vi "3.2.1_BOOST_Air_Muscle_Check.vi"(6 "Data in":T1, 8 "error in (no error)":errorcluster, 9 "AllControls In":T2, 10 "?":T3, 11 "Message Queue out":T4) -> (0 "error out":errorcluster, 1 "Flow":string, 2 "Data":T3, 3 "Message Queue Out":T4, 4 "Data out":T1)   [LabVIEW 2017]
uses:
  Depends/AMC/subVIs/TypeDefs/amc_Message Queue.ctl
  Depends/AMC/subVIs/TypeDefs/amc_Message.ctl
  Depends/Tools/Keyed Array/Tools_KeyedArray KeyedArray.ctl
  Ctrls/Data.ctl
  Ctrls/CSV_Data.ctl
  Ctrls/AllControls.ctl
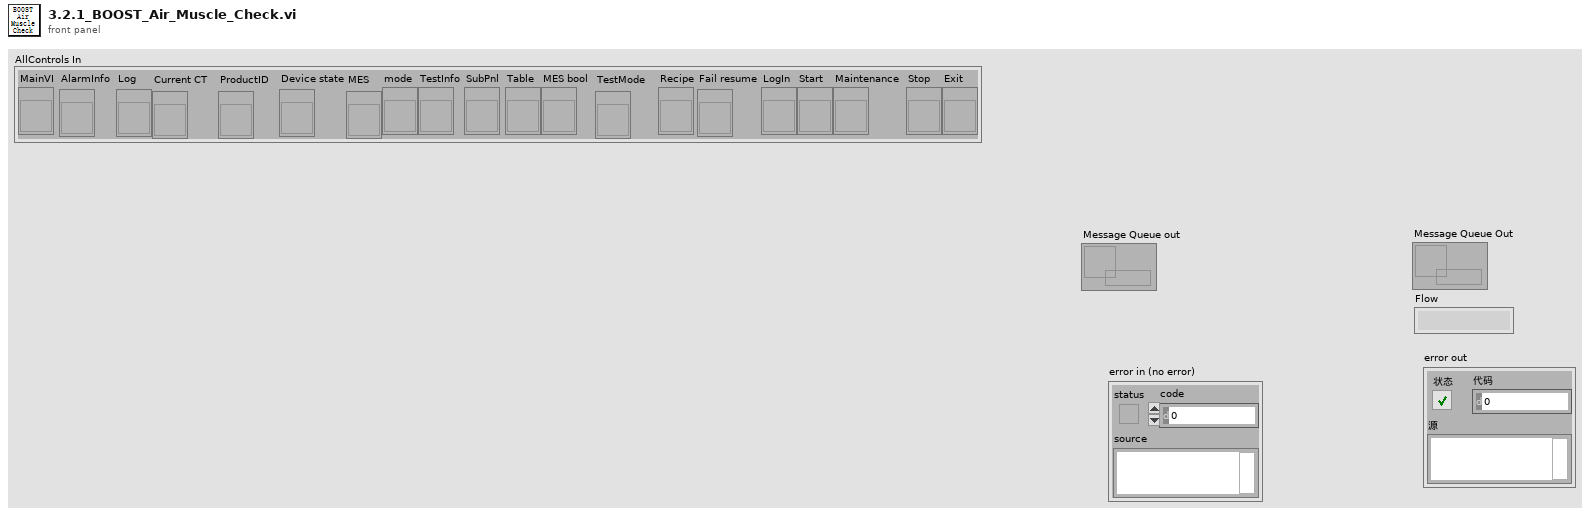
[diagram p1: front panel]
types:
  T1 = typedef "CSV_Data.ctl" = cluster{"Initialisation":cluster{"LMT - Connect UUT (con COM)":string, "LMT - Software Version (rrel)":string, "LMT - Write SKU file (wskuc)":string, "LMT - SKU file name":string, "Connect UUT DDM":string, "Read DDM EOL Timestamp - Mode":string, "Read DDM EOL Timestamp - Timestamp":string, "Read DDM EOL Timestamp - Rig ID":string, "Read DDM EOL Timestamp - Passmark ID":string, "Read DDM EOL Timestamp - Passmark Rev":string, "Software Version before flashing":string, "Read Hardware Serial":string, "UUT DDM SN":string, "Compare DDM SN with MES SN":string, "Backup PCBA Calibration EEPROM Response - CAL":string, "Flash Firmware Version":string, "Check SW Version":string, "Read DDM SW Version after flashing":string, "Set SKU Config":string, "Ready Status":string, "Set Device Mode to EOL":string, "DDM Parameter - Voltage":string, "DDM Parameter - Current":string, "DDM Parameter - Power":string, "DDM Parameter - Speed":string, "DDM Parameter - Pressure":string, "Tester Parameter - Voltage":string, "Tester Parameter - Current":string, "Tester Parameter - Power":string, "Tester Parameter - Ambient Pressure":string, "Tester Parameter - Ambient Temperature":string, "Calculated Parameter - DDM Pressure Corrected":string, "Calculated Parameter - DDM Real Power":string, "Calculated Parameter - Delta V":string}, "BEMF_Calibration":cluster{"Calibration Result - eol_cold_bemf_temp":string, "DDM Ambient Temp":string, "Restriction Plate Diameter":string, "Calibration Result - eol_bemf_mp_cold_coef_a":string, "Calibration Result - eol_bemf_mp_cold_coef_b":string, "Calibration Result - eol_bemf_mp_cold_coef_c":string, "Calibration Result - eol_bemf_lsi_cold_ref_coeffs":string, "Get - Calibration Result - eol_bemf_lsi_speed":string, "Get - Calibration Result - eol_bemf_lsi_integral_0":string, "Calibration Result - eol_bemf_lsi_integral_1":string, "Get - Calibration Result - eol_bemf_lsi_integral_2":string, "Get - Calibration Result - eol_cold_bemf":string, "Get - Calibration Result - eol_cold_bemf_fisf":string, "Finalise Calibration":string, "Compare -Calibration Result - eol_cold_bemf":string, "Compare -Calibration Result - eol_cold_bemf_fisf":string}, "ECO":cluster{"Reset Power Tune":string, "Reset BEMF FISF Calibration":string, "Restriction Plate Diameter":string, "ECO - Stabilisation Time":string, "ECO - DDM Parameter - Voltage":string, "ECO - DDM Parameter - Current":string, "ECO - DDM Parameter - Power":string, "ECO - DDM Parameter - Measured Power":string, "ECO - DDM Parameter - Speed":string, "ECO - DDM Parameter - Pressure":string, "ECO - Tester Parameter - Voltage":string, "ECO - Tester Parameter - Current":string, "ECO - Tester Parameter - Power":string, "ECO - Tester Parameter - Ambient Pressure":string, "ECO - Tester Parameter - Ambient Temperature":string, "ECO - Tester Parameter - Ambient Humidity":string, "ECO - Calculated Parameter - DDM Pressure Corrected":string, "ECO - Calculated Parameter - DDM Real Power":string, "ECO - Calculated Parameter - Delta V":string, "ECO - Calculated Parameter - Flowrate":string, "ECO - Calculated Parameter - Airwatt":string, "ECO - Formula":string, "PT ECO - Power Tune Mode Status":string}, "BOOST":cluster{"Restriction Plate Diameter":string, "BOOST - Stabilisation Time":string, "BOOST - DDM Parameter - Voltage":string, "BOOST - DDM Parameter - Current":string, "BOOST - DDM Parameter - Power":string, "BOOST - DDM Parameter - Measured Power":string, "BOOST - DDM Parameter - Speed":string, "BOOST - DDM Parameter - Pressure":string, "BOOST - Tester Parameter - Voltage":string, "BOOST - Tester Parameter - Current":string, "BOOST - Tester Parameter - Power":string, "BOOST - Tester Parameter - Ambient Pressure":string, "BOOST - Tester Parameter - Ambient Temperature":string, "BOOST - Tester Parameter - Ambient Humidity":string, "BOOST - Calculated Parameter - DDM Pressure Corrected":string, "BOOST - Calculated Parameter - DDM Real Power":string, "BOOST - Calculated Parameter - Delta V":string, "BOOST - Calculated Parameter - Flowrate":string, "BOOST - Calculated Parameter - Airwatt":string, "BOOST - Get AM Presence":string, "Air Muscle Turn Off Status":string, "BOOST - Air Muscle Calculated Parameter - Airwatt B":string, "BOOST - Air Muscle Calculate Airwatt Delta":string, "PT BOOST - Power Tune Mode Status":string, "Finalise Calibration":string, "ECO - Get AW Calibration value":string, "BOOST - Get AW Calibration value":string}, "MAX":cluster{"Restriction Plate Diameter":string, "MAX - Stabilisation Time":string, "Get Average Delta Tmag (LSIdelta_FISFdelta_LSItmag_FISFtmag_IIRtmag)":string, "Get Average Delta Tmag FISF":string, "MAX - DDM Parameter - Voltage":string, "MAX - DDM Parameter - Current":string, "MAX - DDM Parameter - Power":string, "MAX - DDM Parameter - Measured Power":string, "MAX - DDM Parameter - Speed":string, "MAX - DDM Parameter - Pressure":string, "MAX - Tester Parameter - Voltage":string, "MAX - Tester Parameter - Current":string, "MAX - Tester Parameter - Power":string, "MAX - Tester Parameter - Ambient Pressure":string, "MAX - Tester Parameter - Ambient Temperature":string, "MAX - Tester Parameter - Ambient Humidity":string, "MAX - Calculated Parameter - DDM Pressure Corrected":string, "MAX - Calculated Parameter - DDM Real Power":string, "MAX - Calculated Parameter - Delta V":string, "MAX - Calculated Parameter - Flowrate":string, "MAX - Calculated Parameter - Airwatt":string, "MAX_FISF_Check_Average_Delta_Tmag":string, "MAX - FISF - BEMF Finetune Result":string, "MAX tune - Delta P1":string, "MAX tune - Calculated Parameter - Airwatt":string, "Calculate Delta Airwatts - MAX finetune - Delta P2":string, "MAX finetune - DDM Parameter - Voltage":string, "MAX finetune - DDM Parameter - Current":string, "MAX finetune - DDM Parameter - Power":string, "MAX finetune - DDM Parameter - Measured Power":string, "MAX finetune - DDM Parameter - Speed":string, "MAX finetune - DDM Parameter - Pressure":string, "MAX finetune - Tester Parameter - Voltage":string, "MAX finetune - Tester Parameter - Current":string, "MAX finetune - Tester Parameter - Power":string, "MAX finetune - Tester Parameter - Ambient Pressure":string, "MAX finetune - Tester Parameter - Ambient Temperature":string, "MAX finetune - Tester Parameter - Ambient Humidity":string, "MAX finetune - Calculated Parameter - DDM Pressure Corrected":string, "MAX finetune - Calculated Parameter - DDM Real Power":string, "MAX finetune - Calculated Parameter - Delta V":string, "MAX finetune - Calculated Parameter - Flowrate":string, "MAX finetune - Calculated Parameter - Airwatt":string, "Check Derate Result":string, "Delta Tmag FISF":string, "Get Hot BEMF Result":string, "Calculate delta Pressure":string, "Finalise Calibration":string, "Calculate & Check Delta BEMF":string, "Delta P Airwatts Value":string}, "LL":cluster{"DDM Ambient Temp":string, "Restriction Plate Diameter":string, "LL - DDM Parameter - Voltage":string, "LL - DDM Parameter - Current":string, "LL - DDM Parameter - Power":string, "LL - DDM Parameter - Measured Power":string, "LL - DDM Parameter - Speed":string, "LL - DDM Parameter - Pressure":string, "LL - Tester Parameter - Voltage":string, "LL - Tester Parameter - Current":string, "LL - Tester Parameter - Power":string, "LL - DDM Real Power":string, "LL - Calibrate Task Detect LL":string}, "HL":cluster{"HL - DDM Parameter - Voltage":string, "HL - DDM Parameter - Current":string, "HL - DDM Parameter - Power":string, "HL - DDM Parameter - Measured Power":string, "HL - DDM Parameter - Speed":string, "HL - DDM Parameter - Pressure":string, "HL - Tester Parameter - Voltage":string, "HL - Tester Parameter - Current":string, "HL - Tester Parameter - Power":string, "HL - DDM Real Power":string, "HL - Calibrate Task Detect HL":string}, "LH":cluster{"Restriction Plate Diameter":string, "LH - DDM Parameter - Voltage":string, "LH - DDM Parameter - Current":string, "LH - DDM Parameter - Power":string, "LH - DDM Parameter - Measured Power":string, "LH - DDM Parameter - Speed":string, "LH - DDM Parameter - Pressure":string, "LH - Tester Parameter - Voltage":string, "LH - Tester Parameter - Current":string, "LH - Tester Parameter - Power":string, "LH - DDM Real Power":string, "LH - Calibrate Task Detect LH":string}, "HH":cluster{"HH - DDM Parameter - Voltage":string, "HH - DDM Parameter - Current":string, "HH - DDM Parameter - Power":string, "HH - DDM Parameter - Measured Power":string, "HH - DDM Parameter - Speed":string, "HH - DDM Parameter - Pressure":string, "HH - Tester Parameter - Voltage":string, "HH - Tester Parameter - Current":string, "HH - Tester Parameter - Power":string, "HH - DDM Real Power":string, "HH - Calibrate Task Detect HH":string}, "Inlet Blockage Calibration":cluster{"Inlet Blockage Calibration - DDM Parameter - Voltage":string, "Inlet Blockage Calibration - DDM Parameter - Current":string, "Inlet Blockage Calibration - DDM Parameter - Power":string, "Inlet Blockage Calibration - DDM Parameter - Measured Power":string, "Inlet Blockage Calibration - DDM Parameter - Speed":string, "Inlet Blockage Calibration - DDM Parameter - Pressure":string, "Inlet Blockage Calibration - Tester Parameter - Voltage":string, "Inlet Blockage Calibration - Tester Parameter - Current":string, "Inlet Blockage Calibration - Tester Parameter - Power":string, "Inlet Blockage Calibration - DDM Real Power":string, "Calibration Inlet Blockage_E":string, "Finalise Calibration":string, "Get Task Detect LL":string, "Get Task Detect HL":string, "Get Task Detect LH":string, "Get Task Detect HH":string, "Calibration Inlet Blockage":string, "Calibration eol cold bemf temp":string}, "GOOD":cluster{"GOOD UNIT - Clear EEPROM Error Log":string, "GOOD UNIT - Write Product Timestamp - Mode":string, "GOOD UNIT - Write Product Timestamp - Timestamp":string, "GOOD UNIT - Write Product Timestamp - Rig ID":string, "GOOD UNIT - Write Product Timestamp - Passmark ID":string, "GOOD UNIT - Write Product Timestamp - Passmark Rev":string, "GOOD UNIT - Set Device Mode to PROD":string, "GOOD UNIT - Backup PCBA Calibration EEPROM Response":string, "GOOD UNIT - Check Security Bit":string, "GOOD UNIT - Set Calibration Lock":string, "GOOD UNIT - Get_Calibration_Lock":string, "GOOD UNIT - Disconnect UUT":string}, "NG":cluster{"NG UNIT - Read NVM Error":string, "NG UNIT - Set Device Mode to FCT":string, "NG UNIT - Backup PCBA Calibration EEPROM Response - CAL":string, "NG UNIT - Backup PCBA Calibration EEPROM Response - ERROR":string, "NG UNIT - Backup PCBA Calibration EEPROM Response - USAGE":string, "NG UNIT - Disconnect UUT":string}, "SN":string, "Table":string[][], "Count":cluster{"Total":i32, "OK":i32, "NG":i32, "Yield":dbl}, "Start Time":timestamp, "daemon reference":refnum<k5>, "CT":dbl, "Config":string[][], "OK/NG":bool, "Station ID":string, "MES DDM SN":string, "MES PCBA SN":string, "Retest":string, "Lux":string, "Initialisation_Status":cluster{"LMT - Connect UUT (con COM)":string, "LMT - Software Version (rrel)":string, "LMT - Write SKU file (wskuc)":string, "LMT - SKU file name":string, "Connect UUT DDM":string, "Read DDM EOL Timestamp - Mode":string, "Read DDM EOL Timestamp - Timestamp":string, "Read DDM EOL Timestamp - Rig ID":string, "Read DDM EOL Timestamp - Passmark ID":string, "Read DDM EOL Timestamp - Passmark Rev":string, "Software Version before flashing":string, "Read Hardware Serial":string, "UUT DDM SN":string, "Compare DDM SN with MES SN":string, "Backup PCBA Calibration EEPROM Response - CAL":string, "Flash Firmware Version":string, "Check SW Version":string, "Read DDM SW Version after flashing":string, "Set SKU Config":string, "Ready Status":string, "Set Device Mode to EOL":string, "DDM Parameter - Voltage":string, "DDM Parameter - Current":string, "DDM Parameter - Power":string, "DDM Parameter - Speed":string, "DDM Parameter - Pressure":string, "Tester Parameter - Voltage":string, "Tester Parameter - Current":string, "Tester Parameter - Power":string, "Tester Parameter - Ambient Pressure":string, "Tester Parameter - Ambient Temperature":string, "Calculated Parameter - DDM Pressure Corrected":string, "Calculated Parameter - DDM Real Power":string, "Calculated Parameter - Delta V":string}, "BEMF_Calibration_Status":cluster{"Calibration Result - eol_cold_bemf_temp":string, "DDM Ambient Temp":string, "Restriction Plate Diameter":string, "Calibration Result - eol_bemf_mp_cold_coef_a":string, "Calibration Result - eol_bemf_mp_cold_coef_b":string, "Calibration Result - eol_bemf_mp_cold_coef_c":string, "Calibration Result - eol_bemf_lsi_cold_ref_coeffs":string, "Get - Calibration Result - eol_bemf_lsi_speed":string, "Get - Calibration Result - eol_bemf_lsi_integral_0":string, "Calibration Result - eol_bemf_lsi_integral_1":string, "Get - Calibration Result - eol_bemf_lsi_integral_2":string, "Get - Calibration Result - eol_cold_bemf":string, "Get - Calibration Result - eol_cold_bemf_fisf":string, "Finalise Calibration":string, "Compare -Calibration Result - eol_cold_bemf":string, "Compare -Calibration Result - eol_cold_bemf_fisf":string}, "ECO_Status":cluster{"Reset Power Tune":string, "Reset BEMF FISF Calibration":string, "Restriction Plate Diameter":string, "ECO - Stabilisation Time":string, "ECO - DDM Parameter - Voltage":string, "ECO - DDM Parameter - Current":string, "ECO - DDM Parameter - Power":string, "ECO - DDM Parameter - Measured Power":string, "ECO - DDM Parameter - Speed":string, "ECO - DDM Parameter - Pressure":string, "ECO - Tester Parameter - Voltage":string, "ECO - Tester Parameter - Current":string, "ECO - Tester Parameter - Power":string, "ECO - Tester Parameter - Ambient Pressure":string, "ECO - Tester Parameter - Ambient Temperature":string, "ECO - Tester Parameter - Ambient Humidity":string, "ECO - Calculated Parameter - DDM Pressure Corrected":string, "ECO - Calculated Parameter - DDM Real Power":string, "ECO - Calculated Parameter - Delta V":string, "ECO - Calculated Parameter - Flowrate":string, "ECO - Calculated Parameter - Airwatt":string, "ECO - Formula":string, "PT ECO - Power Tune Mode Status":string}, "BOOST_Status":cluster{"Restriction Plate Diameter":string, "BOOST - Stabilisation Time":string, "BOOST - DDM Parameter - Voltage":string, "BOOST - DDM Parameter - Current":string, "BOOST - DDM Parameter - Power":string, "BOOST - DDM Parameter - Measured Power":string, "BOOST - DDM Parameter - Speed":string, "BOOST - DDM Parameter - Pressure":string, "BOOST - Tester Parameter - Voltage":string, "BOOST - Tester Parameter - Current":string, "BOOST - Tester Parameter - Power":string, "BOOST - Tester Parameter - Ambient Pressure":string, "BOOST - Tester Parameter - Ambient Temperature":string, "BOOST - Tester Parameter - Ambient Humidity":string, "BOOST - Calculated Parameter - DDM Pressure Corrected":string, "BOOST - Calculated Parameter - DDM Real Power":string, "BOOST - Calculated Parameter - Delta V":string, "BOOST - Calculated Parameter - Flowrate":string, "BOOST - Calculated Parameter - Airwatt":string, "BOOST - Get AM Presence":string, "Air Muscle Turn Off Status":string, "BOOST - Air Muscle Calculated Parameter - Airwatt B":string, "BOOST - Air Muscle Calculate Airwatt Delta":string, "PT BOOST - Power Tune Mode Status":string, "Finalise Calibration":string, "ECO - Get AW Calibration value":string, "BOOST - Get AW Calibration value":string}, "MAX_Status":cluster{"Restriction Plate Diameter":string, "MAX - Stabilisation Time":string, "Get Average Delta Tmag (LSIdelta_FISFdelta_LSItmag_FISFtmag_IIRtmag)":string, "Get Average Delta Tmag FISF":string, "MAX - DDM Parameter - Voltage":string, "MAX - DDM Parameter - Current":string, "MAX - DDM Parameter - Power":string, "MAX - DDM Parameter - Measured Power":string, "MAX - DDM Parameter - Speed":string, "MAX - DDM Parameter - Pressure":string, "MAX - Tester Parameter - Voltage":string, "MAX - Tester Parameter - Current":string, "MAX - Tester Parameter - Power":string, "MAX - Tester Parameter - Ambient Pressure":string, "MAX - Tester Parameter - Ambient Temperature":string, "MAX - Tester Parameter - Ambient Humidity":string, "MAX - Calculated Parameter - DDM Pressure Corrected":string, "MAX - Calculated Parameter - DDM Real Power":string, "MAX - Calculated Parameter - Delta V":string, "MAX - Calculated Parameter - Flowrate":string, "MAX - Calculated Parameter - Airwatt":string, "MAX_FISF_Check_Average_Delta_Tmag":string, "MAX - FISF - BEMF Finetune Result":string, "MAX tune - Delta P1":string, "MAX tune - Calculated Parameter - Airwatt":string, "Calculate Delta Airwatts - MAX finetune - Delta P2":string, "MAX finetune - DDM Parameter - Voltage":string, "MAX finetune - DDM Parameter - Current":string, "MAX finetune - DDM Parameter - Power":string, "MAX finetune - DDM Parameter - Measured Power":string, "MAX finetune - DDM Parameter - Speed":string, "MAX finetune - DDM Parameter - Pressure":string, "MAX finetune - Tester Parameter - Voltage":string, "MAX finetune - Tester Parameter - Current":string, "MAX finetune - Tester Parameter - Power":string, "MAX finetune - Tester Parameter - Ambient Pressure":string, "MAX finetune - Tester Parameter - Ambient Temperature":string, "MAX finetune - Tester Parameter - Ambient Humidity":string, "MAX finetune - Calculated Parameter - DDM Pressure Corrected":string, "MAX finetune - Calculated Parameter - DDM Real Power":string, "MAX finetune - Calculated Parameter - Delta V":string, "MAX finetune - Calculated Parameter - Flowrate":string, "MAX finetune - Calculated Parameter - Airwatt":string, "Check Derate Result":string, "Delta Tmag FISF":string, "Get Hot BEMF Result":string, "Calculate delta Pressure":string, "Finalise Calibration":string, "Calculate & Check Delta BEMF":string, "Delta P Airwatts Value":string}, "LL_Status":cluster{"DDM Ambient Temp":string, "Restriction Plate Diameter":string, "LL - DDM Parameter - Voltage":string, "LL - DDM Parameter - Current":string, "LL - DDM Parameter - Power":string, "LL - DDM Parameter - Measured Power":string, "LL - DDM Parameter - Speed":string, "LL - DDM Parameter - Pressure":string, "LL - Tester Parameter - Voltage":string, "LL - Tester Parameter - Current":string, "LL - Tester Parameter - Power":string, "LL - DDM Real Power":string, "LL - Calibrate Task Detect LL":string}, "HL_Status":cluster{"HL - DDM Parameter - Voltage":string, "HL - DDM Parameter - Current":string, "HL - DDM Parameter - Power":string, "HL - DDM Parameter - Measured Power":string, "HL - DDM Parameter - Speed":string, "HL - DDM Parameter - Pressure":string, "HL - Tester Parameter - Voltage":string, "HL - Tester Parameter - Current":string, "HL - Tester Parameter - Power":string, "HL - DDM Real Power":string, "HL - Calibrate Task Detect HL":string}, "LH_Status":cluster{"Restriction Plate Diameter":string, "LH - DDM Parameter - Voltage":string, "LH - DDM Parameter - Current":string, "LH - DDM Parameter - Power":string, "LH - DDM Parameter - Measured Power":string, "LH - DDM Parameter - Speed":string, "LH - DDM Parameter - Pressure":string, "LH - Tester Parameter - Voltage":string, "LH - Tester Parameter - Current":string, "LH - Tester Parameter - Power":string, "LH - DDM Real Power":string, "LH - Calibrate Task Detect LH":string}, "HH_Status":cluster{"HH - DDM Parameter - Voltage":string, "HH - DDM Parameter - Current":string, "HH - DDM Parameter - Power":string, "HH - DDM Parameter - Measured Power":string, "HH - DDM Parameter - Speed":string, "HH - DDM Parameter - Pressure":string, "HH - Tester Parameter - Voltage":string, "HH - Tester Parameter - Current":string, "HH - Tester Parameter - Power":string, "HH - DDM Real Power":string, "HH - Calibrate Task Detect HH":string}, "Inlet Blockage Calibration_Status":cluster{"Inlet Blockage Calibration - DDM Parameter - Voltage":string, "Inlet Blockage Calibration - DDM Parameter - Current":string, "Inlet Blockage Calibration - DDM Parameter - Power":string, "Inlet Blockage Calibration - DDM Parameter - Measured Power":string, "Inlet Blockage Calibration - DDM Parameter - Speed":string, "Inlet Blockage Calibration - DDM Parameter - Pressure":string, "Inlet Blockage Calibration - Tester Parameter - Voltage":string, "Inlet Blockage Calibration - Tester Parameter - Current":string, "Inlet Blockage Calibration - Tester Parameter - Power":string, "Inlet Blockage Calibration - DDM Real Power":string, "Calibration Inlet Blockage_E":string, "Finalise Calibration":string, "Get Task Detect LL":string, "Get Task Detect HL":string, "Get Task Detect LH":string, "Get Task Detect HH":string, "Calibration Inlet Blockage":string, "Calibration eol cold bemf temp":string}, "GOOD_Status":cluster{"GOOD UNIT - Clear EEPROM Error Log":string, "GOOD UNIT - Write Product Timestamp - Mode":string, "GOOD UNIT - Write Product Timestamp - Timestamp":string, "GOOD UNIT - Write Product Timestamp - Rig ID":string, "GOOD UNIT - Write Product Timestamp - Passmark ID":string, "GOOD UNIT - Write Product Timestamp - Passmark Rev":string, "GOOD UNIT - Set Device Mode to PROD":string, "GOOD UNIT - Backup PCBA Calibration EEPROM Response":string, "GOOD UNIT - Check Security Bit":string, "GOOD UNIT - Set Calibration Lock":string, "GOOD UNIT - Get_Calibration_Lock":string, "GOOD UNIT - Disconnect UUT":string}, "NG_Status":cluster{"NG UNIT - Read NVM Error":string, "NG UNIT - Set Device Mode to FCT":string, "NG UNIT - Backup PCBA Calibration EEPROM Response - CAL":string, "NG UNIT - Backup PCBA Calibration EEPROM Response - ERROR":string, "NG UNIT - Backup PCBA Calibration EEPROM Response - USAGE":string, "NG UNIT - Disconnect UUT":string}, "SKU":string, "Plate_Diameter":string, "Alarm":string}
  T2 = typedef "AllControls.ctl" = cluster{"MainVI":refnum<vi>, "AlarmInfo":refnum<vi>, "Log":refnum<vi>, "Current CT":refnum<vi>, "ProductID":refnum<vi>, "Device state":refnum<vi>, "MES":refnum<vi>, "mode":refnum<vi>, "TestInfo":refnum<vi>, "SubPnl":refnum<vi>, "Table":refnum<vi>, "MES bool":refnum<vi>, "TestMode":refnum<vi>, "Recipe":refnum<vi>, "Fail resume":refnum<vi>, "LogIn":refnum<vi>, "Start":refnum<vi>, "Maintenance":refnum<vi>, "Stop":refnum<vi>, "Exit":refnum<vi>}
  T3 = typedef "Data.ctl" = cluster{"Initialisation":cluster{"DDM_Parameter":dbl[], "DDM_Parameter_status":bool[], "Get_Tester_Parameter":dbl[], "Get_Tester_Parameter_status":bool[], "Cal_Tester_Parameter":dbl[], "Cal_Tester_Parameter_status":bool[], "sw_version_before_status":bool, "sw_version_after_status":bool, "Set_SKU_Config_With_LMT_status":bool, "FCT_timestamp_status":bool, "LMT_Connect_to_UUT_status":bool}, "BEMF_Calibration":cluster{"Read_ambient_temperature":dbl, "Calibration_Vaule":dbl[], "Calibration_Vaule _B":dbl[], "Calibration_Vaule_status":bool[], "Calibration_Vaule_B_status":bool[]}, "ECO":cluster{"DDM_Parameter":dbl[], "DDM_Parameter_status":bool[], "Get_Tester_Parameter":dbl[], "Get_Tester_Parameter_status":bool[], "Cal_Tester_Parameter":dbl[], "Cal_Tester_Parameter_status":bool[], "DDM_Parameter_after_power_tune":dbl[], "Get_Tester_Parameter_after_power_tune":dbl[], "Cal_Tester_Parameter_after_power_tune":dbl[], "Cal_Tester_Parameter_after_power_tune_status":bool[], "Delta_P":dbl}, "BOOST":cluster{"DDM_Parameter":dbl[], "DDM_Parameter_status":bool[], "Get_Tester_Parameter":dbl[], "Get_Tester_Parameter_status":bool[], "Cal_Tester_Parameter":dbl[], "Cal_Tester_Parameter_status":bool[], "DDM_Parameter_after_power_tune":dbl[], "Get_Tester_Parameter_after_power_tune":dbl[], "Cal_Tester_Parameter_after_power_tune":dbl[], "Cal_Tester_Parameter_after_power_tune_status":bool[], "airwatts_am_off":dbl, "AW_Delta_(AM_on_and_off)":dbl, "AW_Delta_(AM_on_and_off)_Status":bool, "Delta_P":dbl}, "MAX":cluster{"Average_Tmag_Data":cluster{"LSI Delta in degC":dbl, "FISF Delta in degc":dbl, "LSI Tmag in degC":dbl, "Fisf Tmag in degC":dbl, "IIR Tmag in degC":dbl}, "DDM_Parameter":dbl[], "DDM_Parameter_status":bool[], "Get_Tester_Parameter":dbl[], "Get_Tester_Parameter_status":bool[], "Cal_Tester_Parameter":dbl[], "BEMF_Finetune":cluster{"eol_bemf_mp_cold_coef_c":dbl, "eol_cold_bemf_fisf_offset":dbl}, "AW_Tune":cluster{"delta_P1":dbl, "delta_P_Setting":dbl}, "DDM_Parameter_after_Airwatts_Tune":dbl[], "Get_Tester_Parameter_after_Airwatts_Tune":dbl[], "Cal_Tester_Parameter_after_Airwatts_Tune":dbl[], "DDM_Parameter_after_Airwatts_Finetune":dbl[], "Get_Tester_Parameter_after_Airwatts_Finetune":dbl[], "Cal_Tester_Parameter_after_Airwatts_Finetune":dbl[], "AW_Finetune":cluster{"delta_P2":dbl, "delta_P_Setting":dbl}, "Delta_Tmag_after_tune":cluster{"LSI Delta in degC":dbl, "FISF Delta in degc":dbl, "LSI Tmag in degC":dbl, "Fisf Tmag in degC":dbl, "IIR Tmag in degC":dbl}, "Hot Bemf in mV":dbl, "DDM_Pressure":dbl, "Delta_Pressure":dbl, " Cold Bemf in mV":dbl, " delta Bemf":dbl, " delta p":dbl, "Delta_Pressure_status":bool, " delta Bemf_status":bool, "LSI Delta in degC_status":bool, "FISF Delta in degc_status":bool, "Max_check_derate_status_status":bool, "Average_All_data":dbl[][], "Average_Tmag_Data_status":bool[], "Average_Tmag_Data_after_tune_status":bool[], "Cal_Tester_Parameter_status":bool[], "Cal_Tester_Parameter_status_after_Airwatts_Tune":bool[], "Cal_Tester_Parameter_status_after_Airwatts_FineTune":bool[]}, "Task_Detect_Calib":cluster{"LL":cluster{"DDM_Parameter":dbl[], "DDM_Parameter_status":bool[], "Get_Tester_Parameter":dbl[], "Get_Tester_Parameter_status":bool[], "Set_task_detect_A":dbl, "Set_task_detect_A_Status":bool}, "HL":cluster{"DDM_Parameter":dbl[], "DDM_Parameter_status":bool[], "Get_Tester_Parameter":dbl[], "Get_Tester_Parameter_status":bool[], "Set_task_detect_B":dbl, "Set_task_detect_B_Status":bool}, "LH":cluster{"DDM_Parameter":dbl[], "DDM_Parameter_status":bool[], "Get_Tester_Parameter":dbl[], "Get_Tester_Parameter_status":bool[], "Set_task_detect_C":dbl, "Set_task_detect_C_Status":bool}, "HH":cluster{"DDM_Parameter":dbl[], "DDM_Parameter_status":bool[], "Get_Tester_Parameter":dbl[], "Get_Tester_Parameter_status":bool[], "Set_task_detect_D":dbl, "Read_and_check_calibration_Status":bool[], "Set_task_detect_D_Status":bool}, "Get_eol_inlet_blockage_E":dbl, "Calib_vaule":cluster{"Get_task_detect_LL":dbl, "Get_task_detect_HL":dbl, "Get_task_detect_LH":dbl, "Get_task_detect_HH":dbl, "eol_inlet_blockage":dbl, "eol_code_bemf_temp":dbl}, "calibrated temp":dbl, "Inlet_Blockage_Calibration":cluster{"DDM_Parameter":dbl[], "DDM_Parameter_status":bool[], "Get_Tester_Parameter":dbl[], "Get_Tester_Parameter_status":bool[]}, "Get_eol_inlet_blockage_E_Status":bool}, "good":cluster{"Write_Product_TS":cluster{"TIMESTAMP":i64, "RIG_ID":i64, "PASSMARK_ID":i64, "PASSMARK_REV":i64}, "Read_Product_TS":cluster{"TIMESTAMP":i64, "RIG_ID":i64, "PASSMARK_ID":i64, "PASSMARK_REV":i64}, "Good_Check_Secuity_Bit_Stauts":bool}}
  T4 = typedef "amc_Message Queue.ctl" = refnum<queue>
  T5 = typedef "HD Config.ctl" = cluster{" PC":cluster{"PC Address":u8[], "PC Port":i32}, "FCO":cluster{"COM":refnum<visa-resource-name>, "Baudrate":u32}, "DC Power ":cluster{"COM":refnum<visa-resource-name>, "Baudrate":u32}, "PW3336":cluster{"COM":refnum<visa-resource-name>, "Baudrate":u32}, "Lefoo":cluster{"COM":refnum<visa-resource-name>, "Baudrate":u32}, "Tempt&Hum":cluster{"COM":refnum<visa-resource-name>, "Baudrate":u32}, "DIPC":cluster{"COM":refnum<visa-resource-name>}, "Daemon":cluster{"IP Address":string, "Port":u16, "Retry":u16}, "NFC":cluster{"COM":refnum<visa-resource-name>, "Baudrate":u32}, "Fail_resume_mode":bool, "GRR":bool}
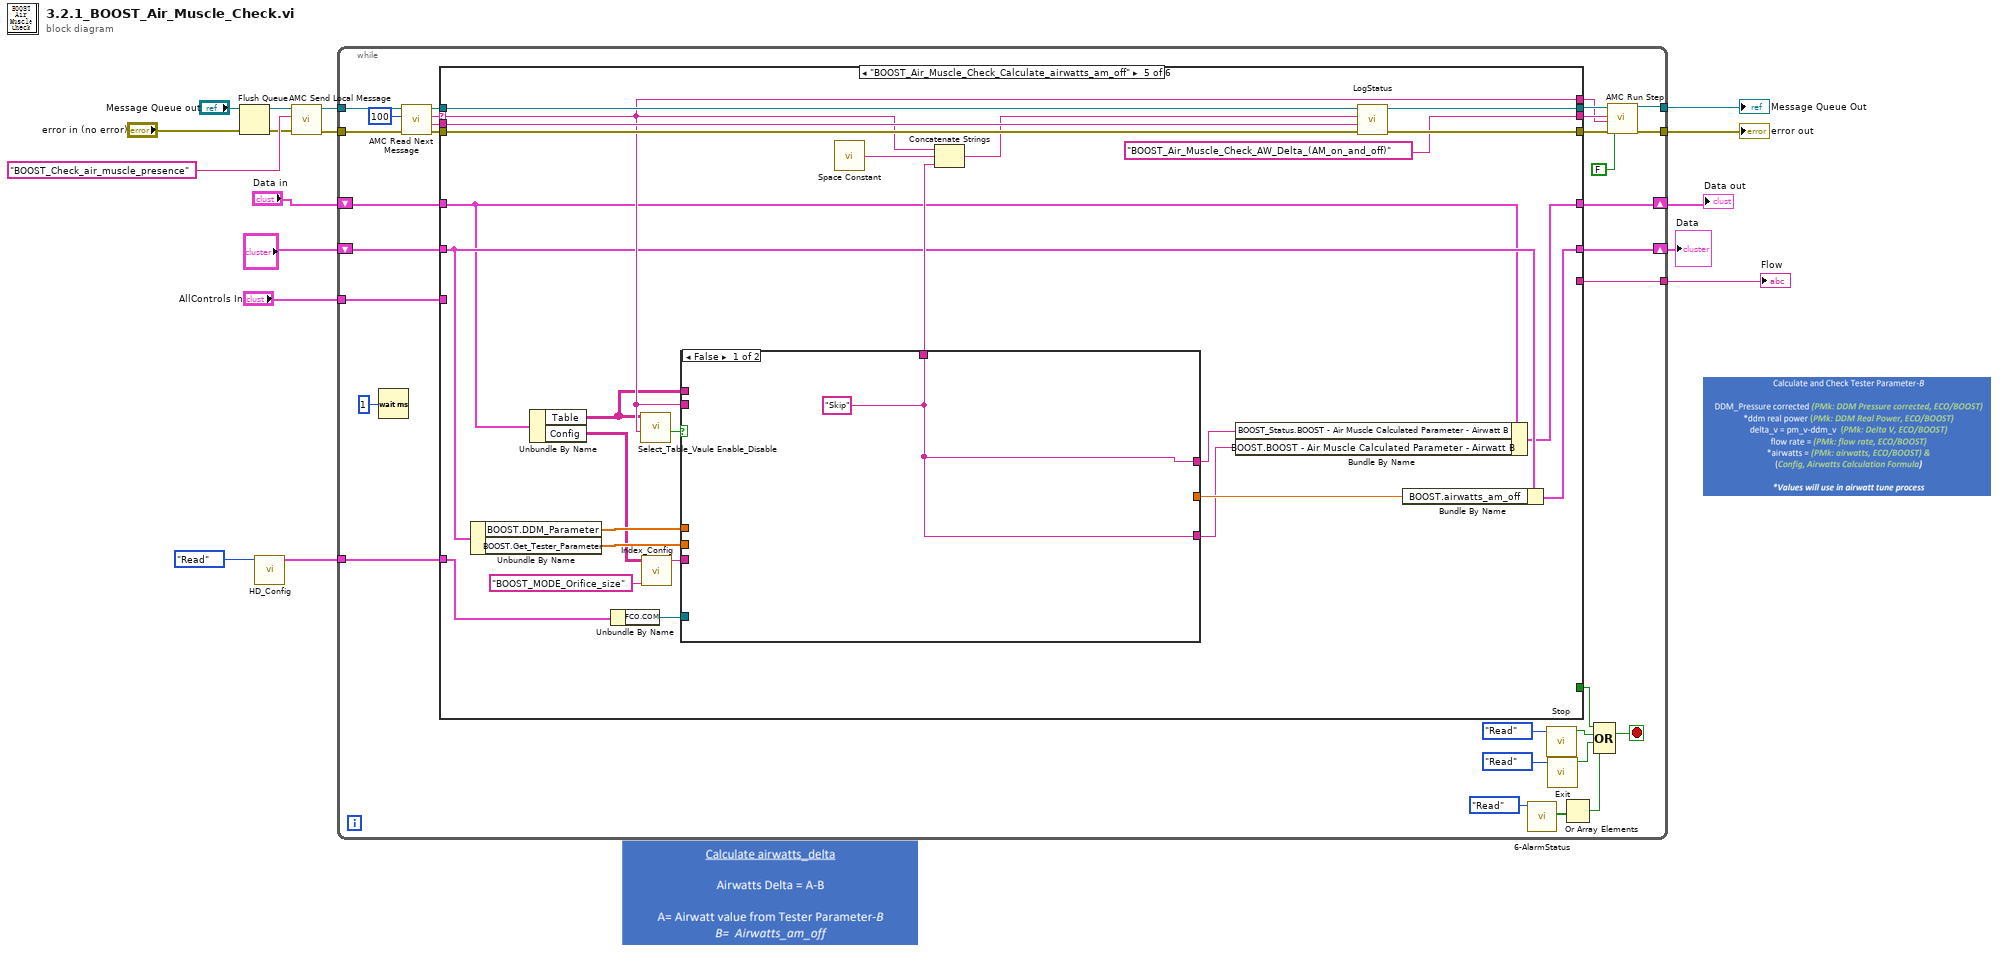
[diagram p0: block diagram]
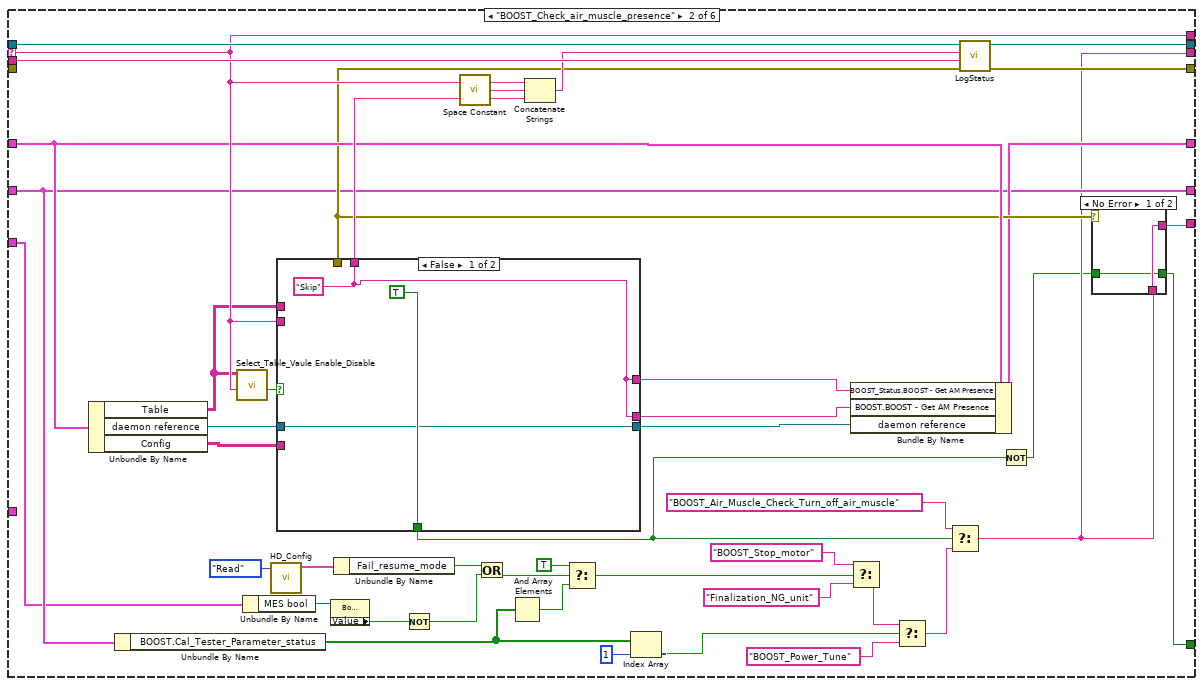
[diagram p3: hidden frame]
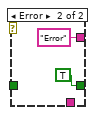
[diagram p4: hidden frame]
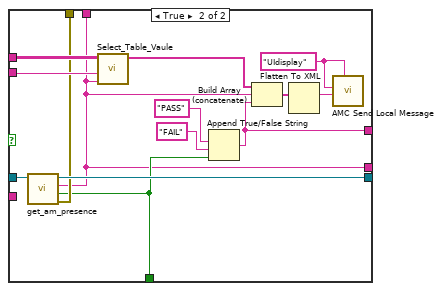
[diagram p5: hidden frame]
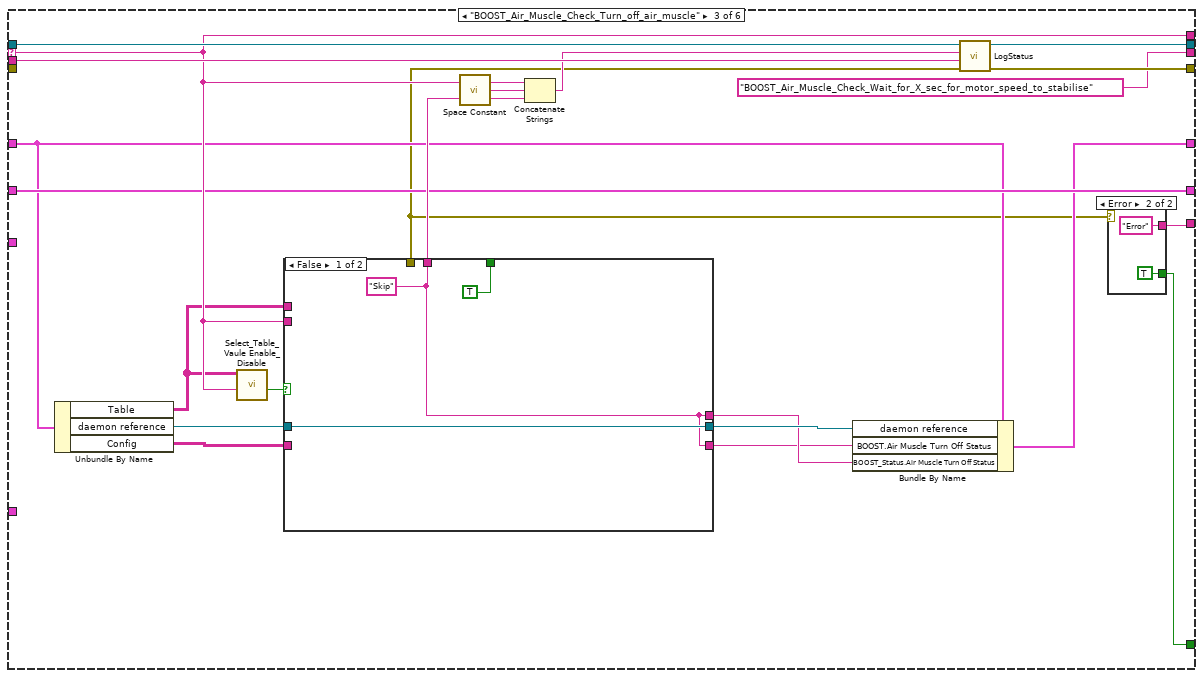
[diagram p6: hidden frame]
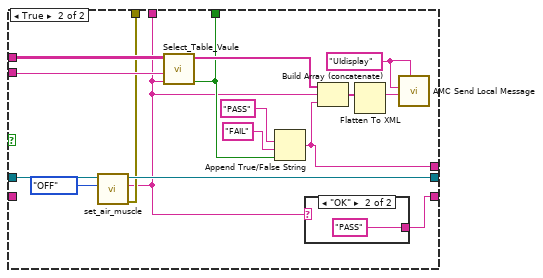
[diagram p8: hidden frame]
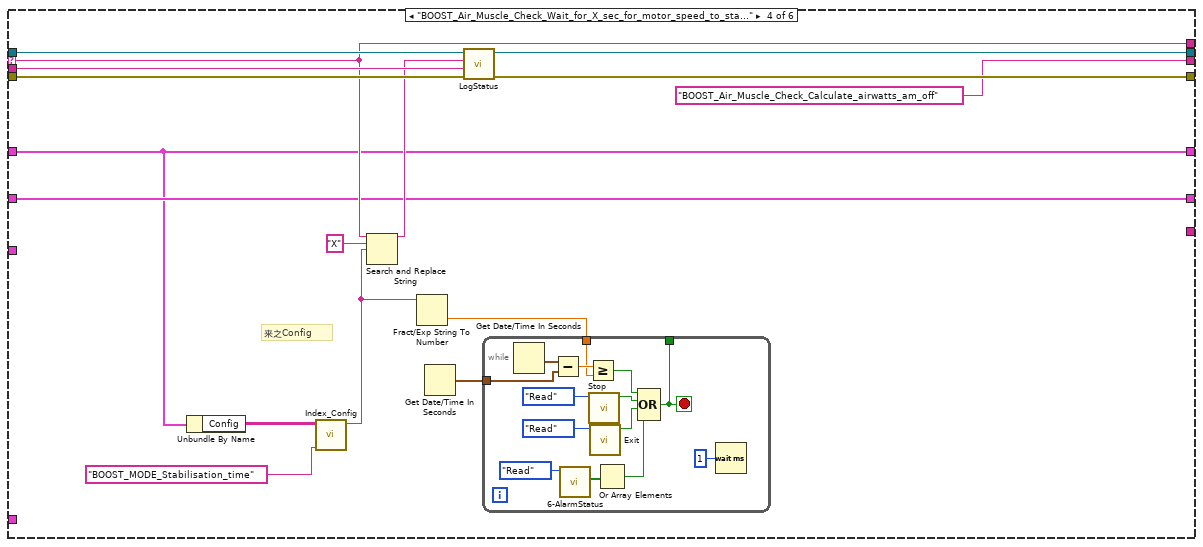
[diagram p10: hidden frame]
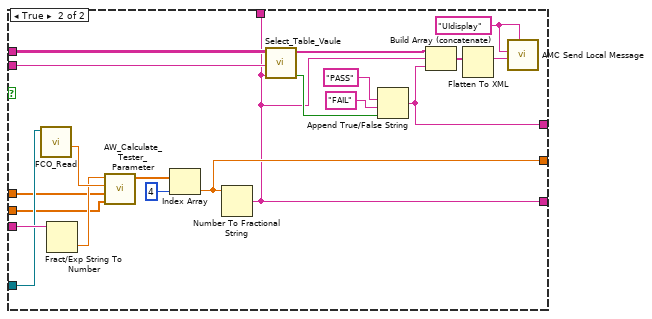
[diagram p11: hidden frame]
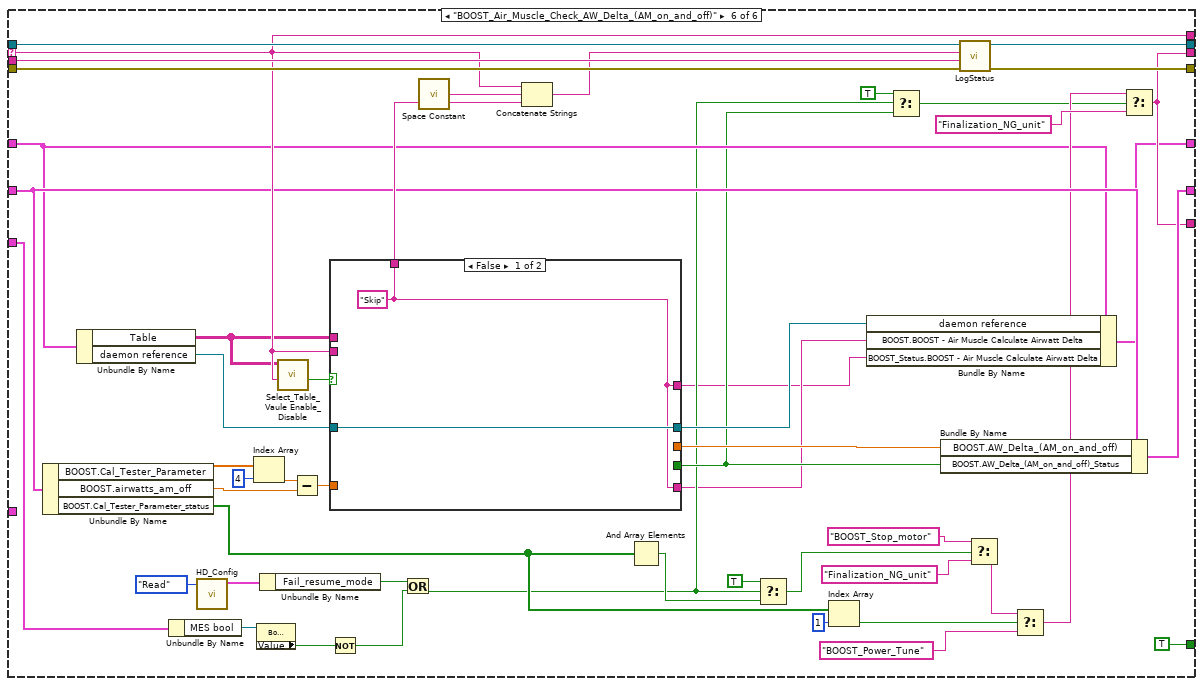
[diagram p12: hidden frame]
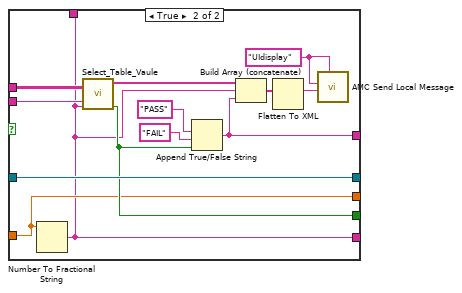
[diagram p13: hidden frame]
diagram:
  n1 = Flush Queue(queue="Message Queue out") -> (queue out=w4:T4)  [unwired: 1 in, 2 out]
  n2 = call "HD_Config.vi"("Step"=enum16{"Initial", "Write", "Read"}."Read") -> ("HD Config out"=w8:T5)  [unwired: 9 in, 1 out]
  n3 = call "AMC Send Local Message.vi"("error in (no error)"="error in (no error)", "Message Name"="BOOST_Check_air_muscle_presence", "Message Queue in"=w4) -> ("error out"=w13:errorcluster, "Message Queue out"=w14:T4)  [unwired: 7 in]
  n4 = while {
    tunnel: w14 -> [w47]
    tunnel: [w43] -> w6
    tunnel: w13 -> [w41]
    tunnel: [w38] -> w5
    shift-right: [w34] -> w10
    shift-left: "?" -> [w35]
    tunnel: w8 -> [w33]
    tunnel: [w29] -> w7
    shift-right: [w21] -> w1
    shift-left: "Data in" -> [w22]
    tunnel: "AllControls In" -> [w20]
    stop <- w23 stop-if-true
    n5 = Wait (ms)(milliseconds to wait=u32 1 ("等待时间（毫秒）")) -> ()  [unwired: 1 out]
    n6 = call "AMC Read Next Message.vi"("error in (no error)"=w41, "timeout (1ms)"=100, "Message Queue in"=w47) -> ("error out"=w40:errorcluster, "Message Value"=w31:string, "Message Name"=w45:string, "Message Queue out"=w46:T4)  [unwired: 1 in, 4 out]
    n7 = case shown="\"BOOST_Air_Muscle_Check_Calculate_airwatts_am_off\"" w45 {
      selector: w45 -> [_ w87 w129 w168 w205 w275]
      tunnel: w46 -> [w51 w94 w136 w174 w213 w283]
      tunnel: [w51 w94 w136 w174 w213 w283] -> w44
      tunnel: w40 -> [w50 _ _ w173 w212 w282]
      tunnel: [w50 w93 w135 w172 w211 w281] -> w39
      tunnel: [_ w83 w125 _ _ TRUE] -> w24
      tunnel: w35 -> [w49 w71 w123 w164 w193 w272]
      tunnel: [w49 w71 w123 w164 w209 w279] -> w34
      tunnel: w31 -> [_ w92 w134 w171 w210 w280]
      tunnel: [_ w87 w129 w168 w205 w275] -> w30
      tunnel: w33 -> [_ _ _ _ w200 _]
      tunnel: [_ w68 "BOOST_Air_Muscle_Check_Wait_for_X_sec_for_motor_speed_to_stabilise" "BOOST_Air_Muscle_Check_Calculate_airwatts_am_off" "BOOST_Air_Muscle_Check_AW_Delta_(AM_on_and_off)" w269] -> w32
      tunnel: [_ w84 w126 _ _ w269] -> w29
      tunnel: w22 -> [w48 w81 w122 w160 w192 w253]
      tunnel: [w48 w79 w119 w160 w191 w252] -> w21
      tunnel: w20 -> [_ w56 _ _ _ w243]
      frame "假", Default {
      }
      frame "BOOST_Check_air_muscle_presence" {
        n8 = Unbundle By Name(w81) -> ("Table"=w86:string[][], "daemon reference"=w91:refnum<k5>, "Config"=w85:string[][])
        n9 = Unbundle By Name(w71) -> ("BOOST.Cal_Tester_Parameter_status"=w70:bool[])
        n10 = call "Select_Table_Vaule Enable_Disable.vi"("Action"=w87, "Table"=w86) -> ("Enable"=w88:bool)  [unwired: 8 in, 1 out]
        n11 = Unbundle By Name(w56) -> ("MES bool"=w60:refnum<vi>)
        n12 = call "HD_Config.vi"("Step"=enum16{"Initial", "Write", "Read"}."Read") -> ("HD Config out"=w59:T5)  [unwired: 9 in, 1 out]
        n13 = case shown="False" w88 {
          tunnel: w91 -> [w100 w107]
          tunnel: [TRUE w104] -> w67
          tunnel: [w100 w106] -> w65
          tunnel: [w99 w103] -> w82
          tunnel: w87 -> [_ w110]
          tunnel: w86 -> [_ w109]
          tunnel: w85 -> [_ _]
          tunnel: [_ w105] -> w80
          tunnel: [w99 w103] -> w53
          tunnel: [w99 w102] -> w52
          frame False {
            w99 = "Skip" ("response")
          }
          frame True {
            w115 = "UIdisplay" ("Process (\"\" - local)")
            n14 = call "get_am_presence.vi"("daemon reference in"=w107) -> ("error out"=w105:errorcluster, "presence?"=w104:bool, "response"=w103:string, "daemon reference out"=w106:refnum<k5>)  [unwired: 6 in, 1 out]
            n15 = call "Select_Table_Vaule.vi"("Vaule"=w103, "Action"=w110, "Table"=w109) -> ("vaule"=w108:string[])  [unwired: 7 in, 1 out]
            n16 = Append True/False String(1:w104, 2:"FAIL" ("真字符串"), 3:"PASS" ("真字符串")) -> (0:w102:string)  [unwired: 1 in]
            n17 = Build Array (concatenate)(w108, w103, w102) -> (w114:string[])
            n18 = Flatten To XML(anything=w114) -> (xml string=w113:string)
            n19 = call "AMC Send Local Message.vi"("Process (\"\" - local)"=w115, "Message Value"=w113, "Message Name"=w115) -> ()  [unwired: 7 in, 2 out]
          }
        }
        n20 = property class="Bool (严格)"(reference=w60) -> ("Value"=w62:bool)  [unwired: 1 in, 2 out]
        n21 = Unbundle By Name(w59) -> ("Fail_resume_mode"=w61:bool)
        n22 = Not(x=w62) -> (.not. x?=w64:bool)
        n23 = call <vilib>:"Space Constant.vi"() -> ("String"=w90:string)
        n24 = Or(x=w61, y=w64) -> (x .or. y?=w63:bool)
        n25 = And Array Elements(Boolean array=w70) -> (logical AND=w55:bool)
        n26 = Concatenate Strings(w87, w90, w82) -> (w89:string)
        n27 = Select(t=TRUE, s=w63, f=w55) -> (s? t:f=w54:bool)
        n28 = Index Array(array=w70, index=1 ("索引")) -> (element=w72:bool)
        n29 = Bundle By Name(cluster=w81, "BOOST_Status.BOOST - Get AM Presence"=w52, "BOOST.BOOST - Get AM Presence"=w53, "daemon reference"=w65) -> (w79:T1)
        n30 = Select(t="BOOST_Stop_motor", s=w54, f="Finalization_NG_unit") -> (s? t:f=w74:string)
        n31 = Select(t=w74, s=w72, f="BOOST_Power_Tune") -> (s? t:f=w69:string)
        n32 = Select(t="BOOST_Air_Muscle_Check_Turn_off_air_muscle" ("Message Name"), s=w67, f=w69) -> (s? t:f=w68:string)
        n33 = call "LogStatus.vi"("error in (no error)"=w80, "last message"=w92, "message"=w89) -> ("error  out"=w93:errorcluster)  [unwired: 8 in]
        n34 = Not(x=w67) -> (.not. x?=w66:bool)
        n35 = case shown="No Error" w80 {
          tunnel: [w95 TRUE] -> w83
          tunnel: [w96 "Error"] -> w84
          tunnel: w68 -> [w96 _]
          tunnel: w66 -> [w95 _]
          frame No Error {
          }
          frame Error {
          }
        }
      }
      frame "BOOST_Air_Muscle_Check_Turn_off_air_muscle" {
        n36 = Unbundle By Name(w122) -> ("Table"=w128:string[][], "daemon reference"=w133:refnum<k5>, "Config"=w127:string[][])
        n37 = call "Select_Table_Vaule Enable_Disable.vi"("Action"=w129, "Table"=w128) -> ("Enable"=w130:bool)  [unwired: 8 in, 1 out]
        n38 = case shown="False" w130 {
          tunnel: w133 -> [w140 w157]
          tunnel: [TRUE w147] -> _
          tunnel: [w140 w151] -> w120
          tunnel: [w139 w143] -> w124
          tunnel: w129 -> [_ w150]
          tunnel: w128 -> [_ w149]
          tunnel: w127 -> [_ _]
          tunnel: [_ w146] -> w118
          tunnel: [w139 w142] -> w116
          tunnel: [w139 w145] -> w117
          frame False {
            w139 = "Skip" ("response")
          }
          frame True {
            w156 = "UIdisplay" ("Process (\"\" - local)")
            n39 = call "set_air_muscle.vi"("control"=enum16{"OFF", "ON", "DISABLE"}."OFF", "daemon reference in"=w157) -> ("error out"=w146:errorcluster, "response"=w143:string, "daemon reference out"=w151:refnum<k5>)  [unwired: 6 in, 1 out]
            n40 = call "Select_Table_Vaule.vi"("Vaule"=w143, "Action"=w150, "Table"=w149) -> ("Result"=w147:bool, "vaule"=w148:string[])  [unwired: 7 in]
            n41 = Append True/False String(1:w147, 2:"FAIL" ("真字符串"), 3:"PASS" ("真字符串")) -> (0:w145:string)  [unwired: 1 in]
            n42 = case shown="\"OK\"" w143 {
              selector: w143 -> [w158 _]
              tunnel: [w158 "PASS"] -> w142
              frame "假", Default {
              }
              frame "OK" {
              }
            }
            n43 = Build Array (concatenate)(w148, w143, w145) -> (w155:string[])
            n44 = Flatten To XML(anything=w155) -> (xml string=w154:string)
            n45 = call "AMC Send Local Message.vi"("Process (\"\" - local)"=w156, "Message Value"=w154, "Message Name"=w156) -> ()  [unwired: 7 in, 2 out]
          }
        }
        n46 = call <vilib>:"Space Constant.vi"() -> ("String"=w132:string)
        n47 = Concatenate Strings(w129, w132, w124) -> (w131:string)
        n48 = Bundle By Name(cluster=w122, "daemon reference"=w120, "BOOST.Air Muscle Turn Off Status"=w116, "BOOST_Status.Air Muscle Turn Off Status"=w117) -> (w119:T1)
        n49 = call "LogStatus.vi"("error in (no error)"=w118, "last message"=w134, "message"=w131) -> ("error  out"=w135:errorcluster)  [unwired: 8 in]
        n50 = case shown="Error" w118 {
          tunnel: [_ TRUE] -> w125
          tunnel: [_ "Error"] -> w126
          frame No Error {
          }
          frame Error {
          }
        }
      }
      frame "BOOST_Air_Muscle_Check_Wait_for_X_sec_for_motor_speed_to_stabilise" {
        # "来之Config"
        n51 = Unbundle By Name(w160) -> ("Config"=w166:string[][])
        n52 = call "Index_Config.vi"("Action"="BOOST_MODE_Stabilisation_time", "config"=w166) -> ("data"=w163:string)  [unwired: 9 in]
        n53 = Search and Replace String(input string=w168, search string="X" ("搜索字符串"), replace string=w163) -> (result string=w167:string)  [unwired: 5 in, 3 out]
        n54 = Fract/Exp String To Number(string=w163) -> (number=w161:dbl)  [unwired: 3 in, 1 out]
        n55 = Get Date/Time In Seconds() -> (seconds since 1Jan1904=w162:timestamp)
        n56 = call "LogStatus.vi"("error in (no error)"=w173, "last message"=w171, "message"=w167) -> ("error  out"=w172:errorcluster)  [unwired: 8 in]
        n57 = while {
          tunnel: w162 -> [w181]
          tunnel: w161 -> [w178]
          tunnel: [w177] -> _
          stop <- w177 stop-if-true
          n58 = Get Date/Time In Seconds() -> (seconds since 1Jan1904=w182:timestamp)
          n59 = Subtract(x=w182, y=w181) -> (x-y=w180:dbl)
          n60 = call "6-AlarmStatus.vi"("Step"=enum16{"Initial", "Write", "Read"}."Read") -> ("AlarmValue Out"=w185:bool[])  [unwired: 9 in, 1 out]
          n61 = Greater Or Equal?(x=w180, y=w178) -> (x >= y?=w179:bool)
          n62 = call "Stop.vi"("Step"=enum16{"Initial", "Write", "Read"}."Read") -> ("Stop Out"=w183:bool)  [unwired: 9 in, 1 out]
          n63 = call "Exit.vi"("Step"=enum16{"Initial", "Write", "Read"}."Read" ("step")) -> ("Exit Out"=w187:bool)  [unwired: 9 in, 1 out]
          n64 = Or Array Elements(Boolean array=w185) -> (logical OR=w184:bool)
          n65 = Compound Arithmetic op=OR(w179, w183, w187, w184) -> (w177:bool)
          n66 = Wait (ms)(milliseconds to wait=u32 1 ("等待时间（毫秒）")) -> ()  [unwired: 1 out]
        }
      }
      frame "BOOST_Air_Muscle_Check_Calculate_airwatts_am_off" {
        n67 = Unbundle By Name(w193) -> ("BOOST.DDM_Parameter"=w197:dbl[], "BOOST.Get_Tester_Parameter"=w196:dbl[])
        n68 = Unbundle By Name(w192) -> ("Table"=w195:string[][], "Config"=w194:string[][])
        n69 = Unbundle By Name(w200) -> ("FCO.COM"=w198:refnum<visa-resource-name>)
        n70 = call "Select_Table_Vaule Enable_Disable.vi"("Action"=w205, "Table"=w195) -> ("Enable"=w204:bool)  [unwired: 8 in, 1 out]
        n71 = call "Index_Config.vi"("Action"="BOOST_MODE_Orifice_size", "config"=w194) -> ("data"=w199:string)  [unwired: 9 in]
        n72 = case shown="False" w204 {
          tunnel: [w214 w215] -> w206
          tunnel: w205 -> [_ w232]
          tunnel: w195 -> [_ w234]
          tunnel: [_ w218] -> w202
          tunnel: w199 -> [_ w223]
          tunnel: w198 -> [_ w222]
          tunnel: w197 -> [_ w221]
          tunnel: w196 -> [_ w220]
          tunnel: [w214 w216] -> w189
          tunnel: [w214 w215] -> w190
          frame False {
            w214 = "Skip" ("software string")
          }
          frame True {
            w231 = "UIdisplay" ("Process (\"\" - local)")
            n73 = call "FCO_Read.vi"("VISA in"=w222) -> ("Pressure(Pa)"=w225:dbl)  [unwired: 7 in, 3 out]
            n74 = Fract/Exp String To Number(string=w223) -> (number=w224:dbl)  [unwired: 3 in, 1 out]
            n75 = call "AW_Calculate_Tester_Parameter.vi"("Tester Parameter"=w220, "DDM Parameter"=w221, "AW_Box_Pressure/Stag Total-Static Pressure rise"=w225, "Orifice_Plate_Diameter"=w224) -> ("Calculate Tester Parameter"=w219:dbl[])  [unwired: 7 in]
            n76 = Index Array(array=w219, index=4) -> (element=w218:dbl)
            n77 = Number To Fractional String(number=w218) -> (F-format string=w215:string)  [unwired: 3 in]
            n78 = call "Select_Table_Vaule.vi"("Vaule"=w215, "Action"=w232, "Table"=w234) -> ("Result"=w233:bool, "vaule"=w226:string[])  [unwired: 7 in]
            n79 = Append True/False String(1:w233, 2:"FAIL" ("真字符串"), 3:"PASS" ("真字符串")) -> (0:w216:string)  [unwired: 1 in]
            n80 = Build Array (concatenate)(w226, w215, w216) -> (w230:string[])
            n81 = Flatten To XML(anything=w230) -> (xml string=w229:string)
            n82 = call "AMC Send Local Message.vi"("Process (\"\" - local)"=w231, "Message Value"=w229, "Message Name"=w231) -> ()  [unwired: 7 in, 2 out]
          }
        }
        n83 = call <vilib>:"Space Constant.vi"() -> ("String"=w208:string)
        n84 = Concatenate Strings(w205, w208, w206) -> (w207:string)
        n85 = Bundle By Name(cluster=w192, "BOOST_Status.BOOST - Air Muscle Calculated Parameter - Airwatt B"=w189, "BOOST.BOOST - Air Muscle Calculated Parameter - Airwatt B"=w190) -> (w191:T1)
        n86 = call "LogStatus.vi"("error in (no error)"=w212, "last message"=w210, "message"=w207) -> ("error  out"=w211:errorcluster)  [unwired: 8 in]
        n87 = Bundle By Name(cluster=w193, "BOOST.airwatts_am_off"=w202) -> (w209:T3)
      }
      frame "BOOST_Air_Muscle_Check_AW_Delta_(AM_on_and_off)" {
        n88 = Unbundle By Name(w272) -> ("BOOST.Cal_Tester_Parameter"=w268:dbl[], "BOOST.airwatts_am_off"=w265:dbl, "BOOST.Cal_Tester_Parameter_status"=w257:bool[])
        n89 = Unbundle By Name(w253) -> ("Table"=w255:string[][], "daemon reference"=w254:refnum<k5>)
        n90 = Unbundle By Name(w243) -> ("MES bool"=w249:refnum<vi>)
        n91 = call "HD_Config.vi"("Step"=enum16{"Initial", "Write", "Read"}."Read") -> ("HD Config out"=w250:T5)  [unwired: 9 in, 1 out]
        n92 = Index Array(array=w268, index=4 ("索引")) -> (element=w266:dbl)
        n93 = property class="Bool (严格)"(reference=w249) -> ("Value"=w247:bool)  [unwired: 1 in, 2 out]
        n94 = Unbundle By Name(w250) -> ("Fail_resume_mode"=w248:bool)
        n95 = call "Select_Table_Vaule Enable_Disable.vi"("Action"=w275, "Table"=w255) -> ("Enable"=w274:bool)  [unwired: 8 in, 1 out]
        n96 = Subtract(x=w266, y=w265) -> (x-y=w264:dbl)
        n97 = case shown="False" w274 {
          tunnel: w254 -> [w285 w297]
          tunnel: [w285 w297] -> w251
          tunnel: [w284 w287] -> w276
          tunnel: w275 -> [_ w295]
          tunnel: w255 -> [_ w298]
          tunnel: [_ w288] -> w273
          tunnel: [_ w296] -> w238
          tunnel: w264 -> [_ w288]
          tunnel: [w284 w287] -> w236
          tunnel: [w284 w286] -> w235
          frame False {
            w284 = "Skip" ("software string")
          }
          frame True {
            w294 = "UIdisplay" ("Process (\"\" - local)")
            n98 = Number To Fractional String(number=w288) -> (F-format string=w287:string)  [unwired: 3 in]
            n99 = call "Select_Table_Vaule.vi"("Vaule"=w287, "Action"=w295, "Table"=w298) -> ("Result"=w296:bool, "vaule"=w289:string[])  [unwired: 7 in]
            n100 = Append True/False String(1:w296, 2:"FAIL" ("真字符串"), 3:"PASS" ("真字符串")) -> (0:w286:string)  [unwired: 1 in]
            n101 = Build Array (concatenate)(w289, w287, w286) -> (w293:string[])
            n102 = Flatten To XML(anything=w293) -> (xml string=w292:string)
            n103 = call "AMC Send Local Message.vi"("Process (\"\" - local)"=w294, "Message Value"=w292, "Message Name"=w294) -> ()  [unwired: 7 in, 2 out]
          }
        }
        n104 = Not(x=w247) -> (.not. x?=w246:bool)
        n105 = Or(x=w248, y=w246) -> (x .or. y?=w237:bool)
        n106 = call <vilib>:"Space Constant.vi"() -> ("String"=w278:string)
        n107 = Concatenate Strings(w275, w278, w276) -> (w277:string)
        n108 = And Array Elements(Boolean array=w257) -> (logical AND=w242:bool)
        n109 = Select(t=TRUE, s=w237, f=w242) -> (s? t:f=w241:bool)
        n110 = Index Array(array=w257, index=1 ("索引")) -> (element=w258:bool)
        n111 = Bundle By Name(cluster=w253, "daemon reference"=w251, "BOOST.BOOST - Air Muscle Calculate Airwatt Delta"=w236, "BOOST_Status.BOOST - Air Muscle Calculate Airwatt Delta"=w235) -> (w252:T1)
        n112 = Select(t=TRUE, s=w237, f=w238) -> (s? t:f=w239:bool)
        n113 = Bundle By Name(cluster=w272, "BOOST.AW_Delta_(AM_on_and_off)"=w273, "BOOST.AW_Delta_(AM_on_and_off)_Status"=w238) -> (w279:T3)
        n114 = call "LogStatus.vi"("error in (no error)"=w282, "last message"=w280, "message"=w277) -> ("error  out"=w281:errorcluster)  [unwired: 8 in]
        n115 = Select(t="BOOST_Stop_motor", s=w241, f="Finalization_NG_unit") -> (s? t:f=w260:string)
        n116 = Select(t=w260, s=w258, f="BOOST_Power_Tune") -> (s? t:f=w256:string)
        n117 = Select(t=w256, s=w239, f="Finalization_NG_unit") -> (s? t:f=w269:string)
      }
    }
    n118 = call "6-AlarmStatus.vi"("Step"=enum16{"Initial", "Write", "Read"}."Read") -> ("AlarmValue Out"=w18:bool[])  [unwired: 9 in, 1 out]
    n119 = call "Stop.vi"("Step"=enum16{"Initial", "Write", "Read"}."Read") -> ("Stop Out"=w26:bool)  [unwired: 9 in, 1 out]
    n120 = call "Exit.vi"("Step"=enum16{"Initial", "Write", "Read"}."Read" ("step")) -> ("Exit Out"=w25:bool)  [unwired: 9 in, 1 out]
    n121 = Or Array Elements(Boolean array=w18) -> (logical OR=w17:bool)
    n122 = Compound Arithmetic op=OR(w24, w26, w25, w17) -> (w23:bool)
    n123 = call "AMC Run Step.vi"("Message Queue In"=w44, "Message Name"=w32, "Message Value"=w30, "error in (no error)"=w39, "Mli/Sig"=FALSE) -> ("Message Queue Out"=w43:T4, "error out"=w38:errorcluster)  [unwired: 13 in]
  }
  "Message Queue Out" <- w6
  "error out" <- w5
  "Data" <- w10
  "Flow" <- w7
  "Data out" <- w1
